vi "TestDataBase_1.vi"(9 "TableName":string="TestTable1", 10 "Select":string(combo)="Idle") -> (3 "ReadData":string[][](array[string]))   [LabVIEW 2024]
uses:
  Controls/Data_Cluster_TestDataBase.ctl
  Controls/DataBaseControl_Test.ctl
  <vilib>/addons/database/Auxilliary.llb/DB Tools Column Info.ctl
  <vilib>/addons/database/Auxilliary.llb/DB Tools DataTypes.ctl
  <vilib>/addons/database/Connection.llb/DB Tools Open Connec (String).vi
  <vilib>/addons/database/_DB Variant To Data/Database Variant To Data.xnode
  <vilib>/addons/database/NI_Database_API.lvlib
panel:
  out "time string":string
  out "date string":string
  out "concatenated string 2":string
  out "Select 2":string
  out "array":string[](array[string])
  out "String 2":string
  in  "Tab Control 2":enum32{"Page 1", "Page 2"}(tab)
  in  "BARCODE":string="1111"
  in  "Tab Control":enum32{"Page 1", "Page 2"}(tab)
  in  "Station4":T1={"BarCode"="1111", "Data1"="10", "Data2"="11", "Data3"="12"}
  in  "Station3":T1={"BarCode"="1111", "Data1"="7", "Data2"="8", "Data3"="9"}
  in  "Station2":T1={"BarCode"="1111", "Data1"="4", "Data2"="6", "Data3"="6"}
  in  "Station1":T1={"BarCode"="1112", "Data1"="1", "Data2"="2", "Data3"="3"}
  out "Date_Time":cluster{"Date":string, "Time":string}
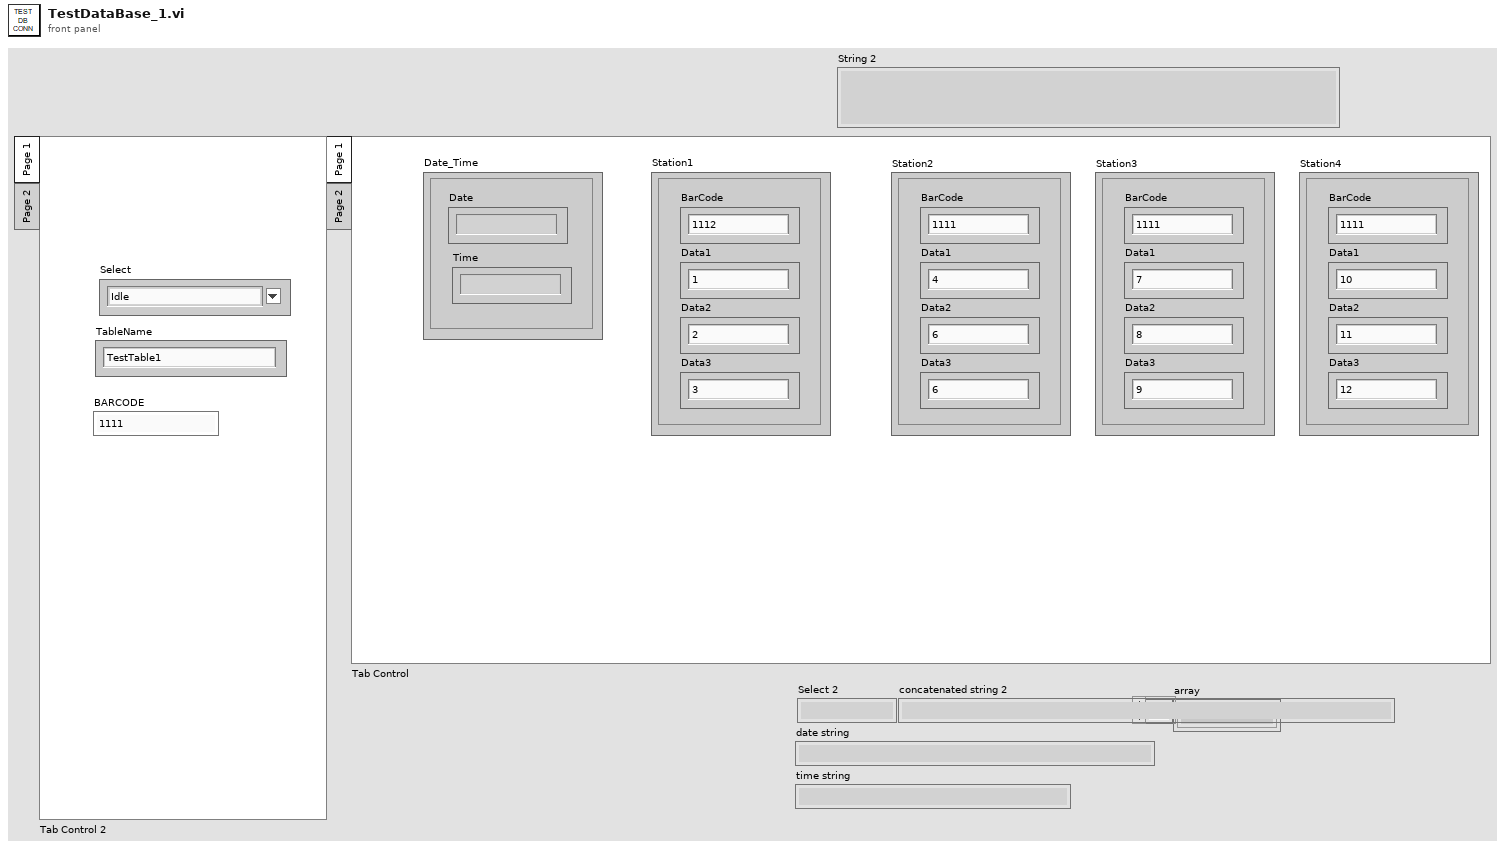
[diagram p1: front panel]
types:
  T1 = typedef "Data_Cluster_TestDataBase.ctl" = cluster{"BarCode":string, "Data1":string, "Data2":string, "Data3":string}
  T2 = typedef "DataBaseControl_Test.ctl" = cluster{"Date_Time":cluster{"Date":string, "Time":string}, "Station1":T1, "Station2":T1, "Station3":T1, "Station4":T1, "BARCODE":string, "ReadData":string[][]}
  T3 = typedef "NI_Database_API.lvlib/DB Tools Column Info.ctl" = cluster{"column name":string, "data type":T4, "size":i32, "allow null?":bool}
  T4 = typedef "NI_Database_API.lvlib/DB Tools DataTypes.ctl" = enum16{"String", "Long (I32)", "Single (SGL)", "Double (DBL)", "Date/Time", "Binary"}
  T5 = typedef "NI_Database_API.lvlib/Conn ObjectReference.ctl" = refnum<k1>
  T6 = cluster{"[0]":string, "[1]":string, "[2]":string, "[3]":string, "[4]":string, "[5]":string, "[6]":string, "[7]":string, "[8]":string, "[9]":string, "[10]":string, "[11]":string, "[12]":string, "[13]":string, "[14]":string, "[15]":string, "[16]":string, "[17]":string}
  T7 = cluster{"output array[0]":string, "output array[1]":string, "output array[2]":string, "output array[3]":string, "output array[4]":string, "output array[5]":string, "output array[6]":string, "output array[7]":string, "output array[8]":string, "output array[9]":string, "output array[10]":string, "output array[11]":string, "output array[12]":string, "output array[13]":string, "output array[14]":string, "output array[15]":string, "output array[16]":string, "output array[17]":string}
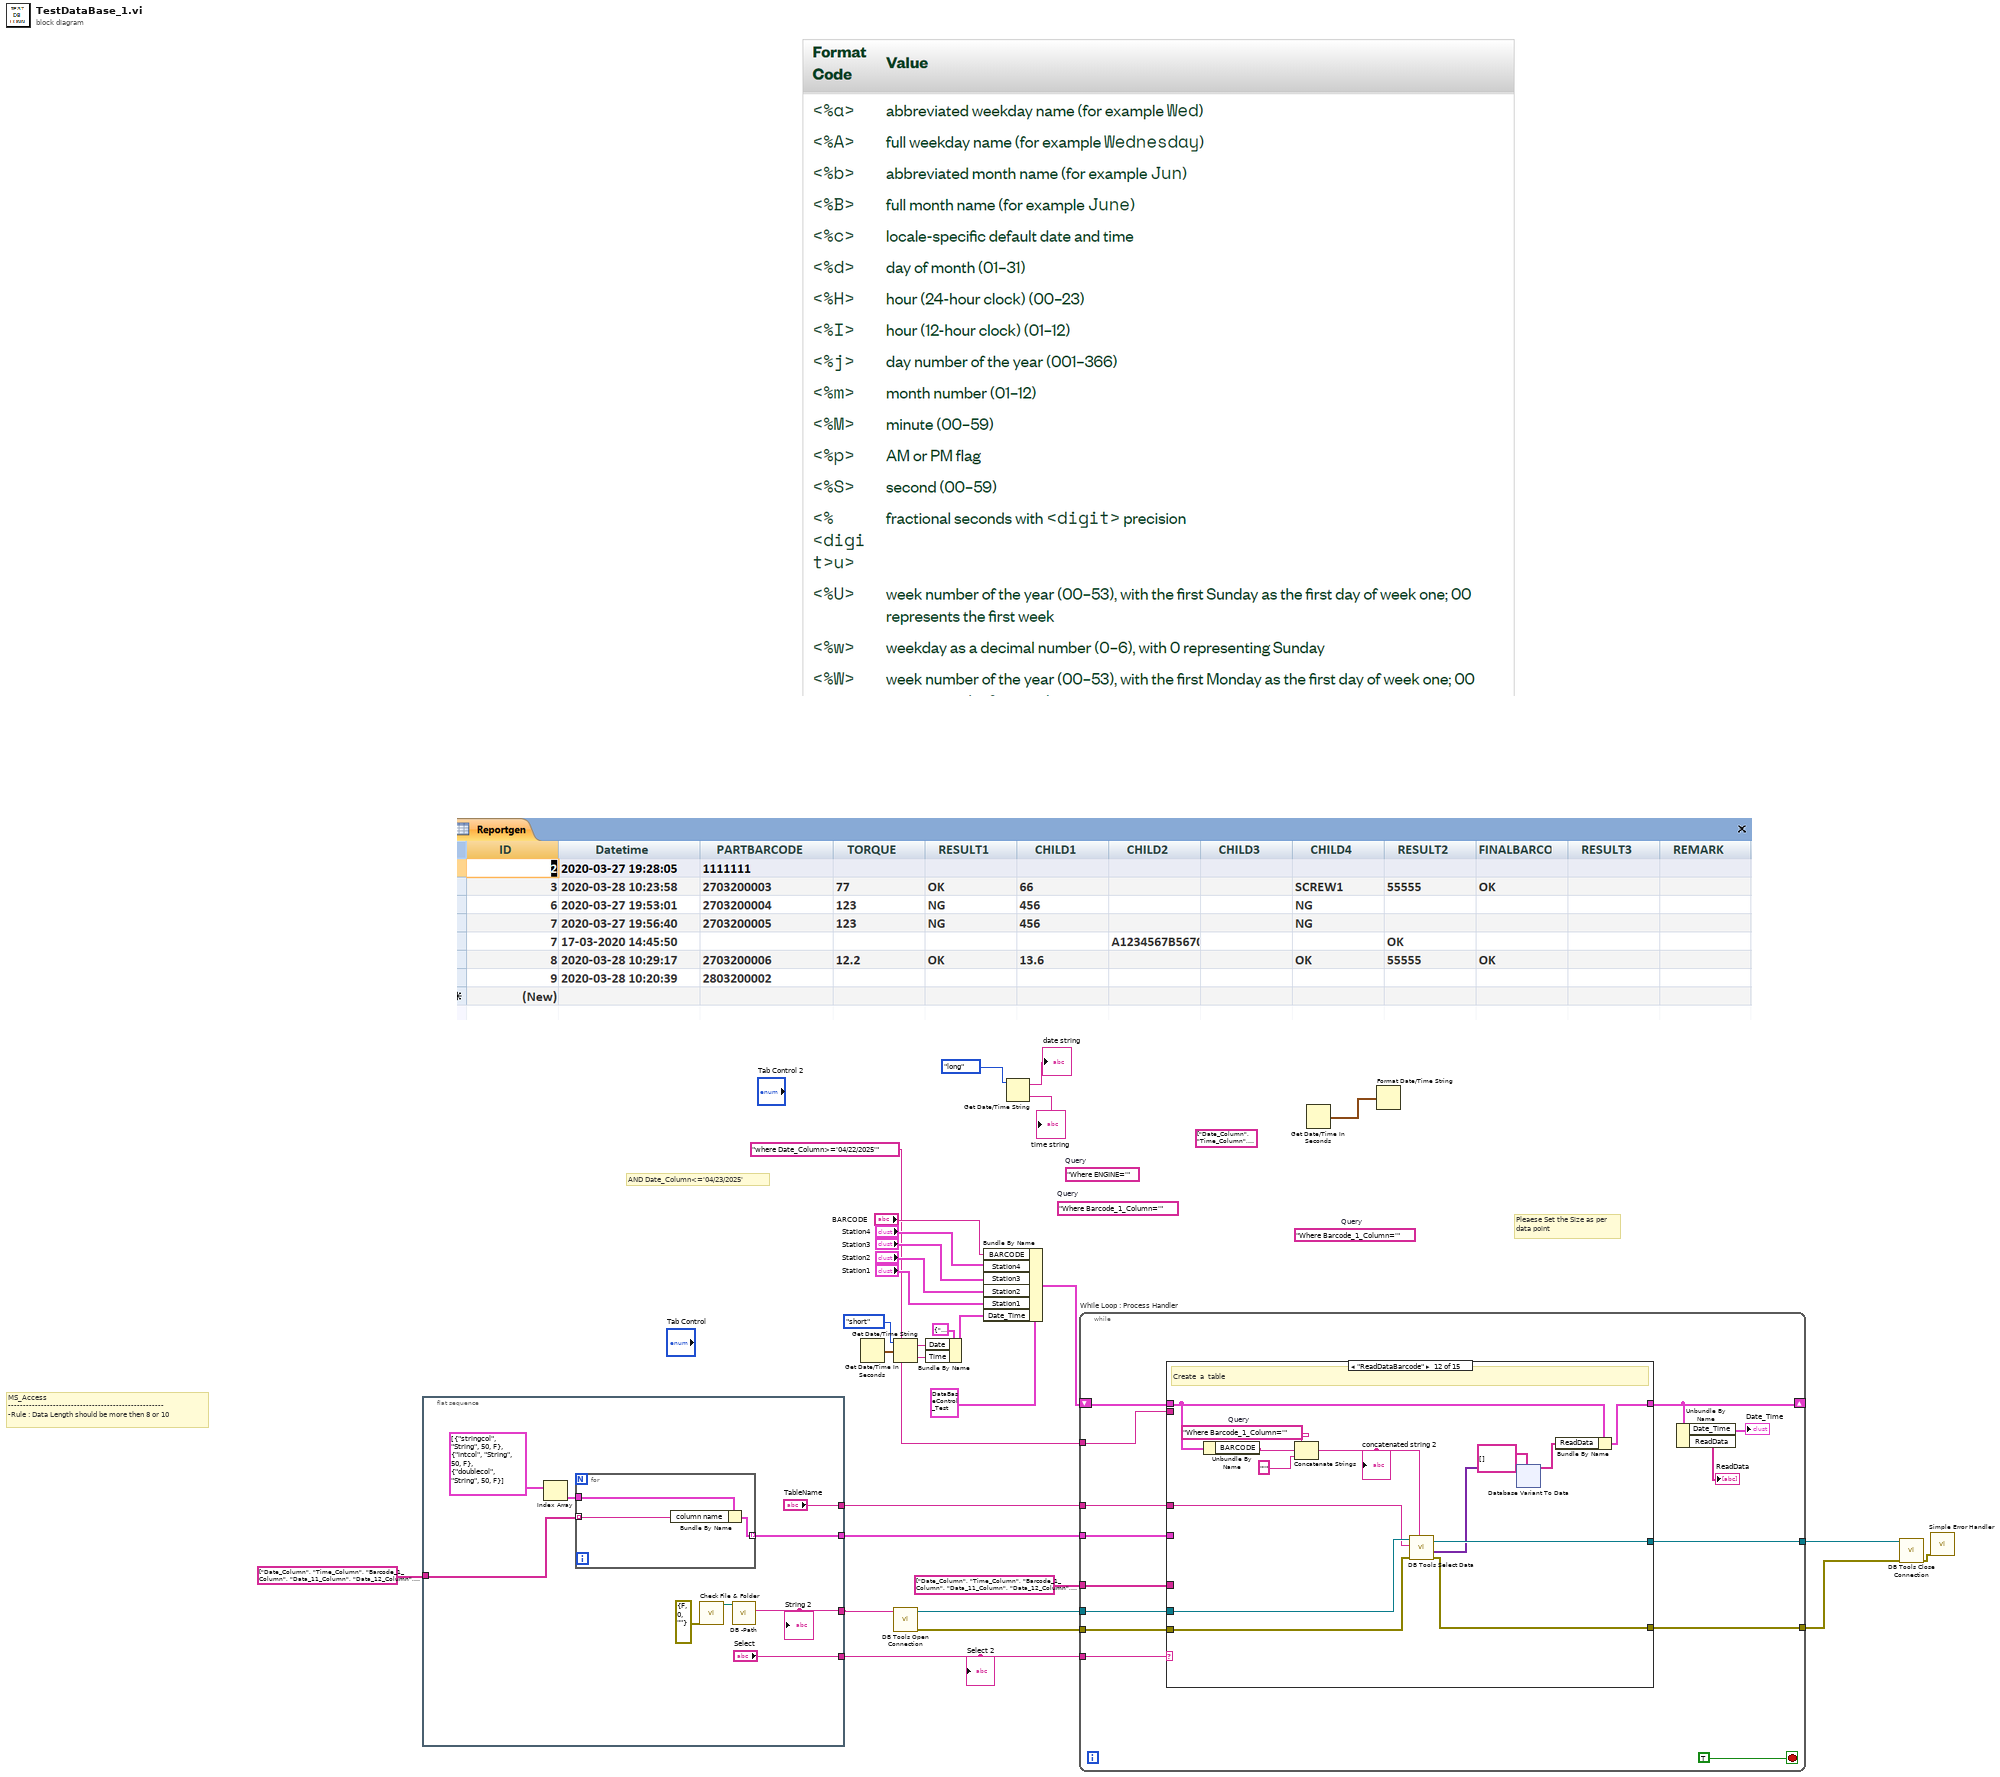
[diagram p0: block diagram]
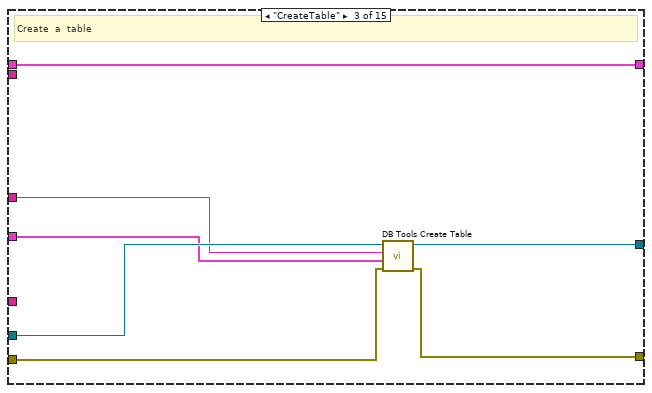
[diagram p4: hidden frame]
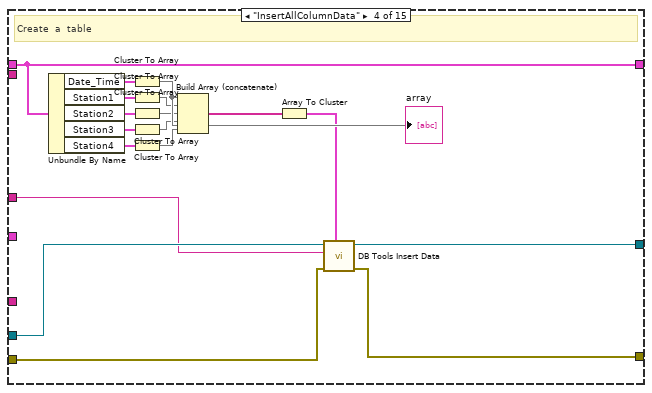
[diagram p5: hidden frame]
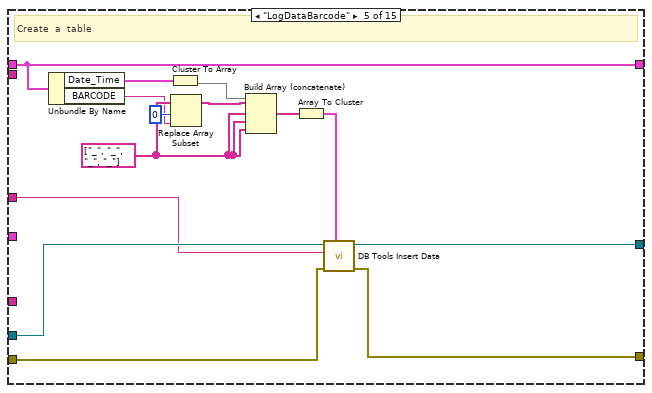
[diagram p6: hidden frame]
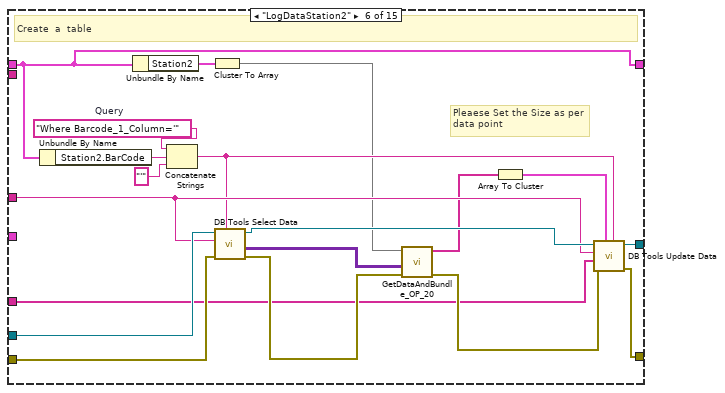
[diagram p7: hidden frame]
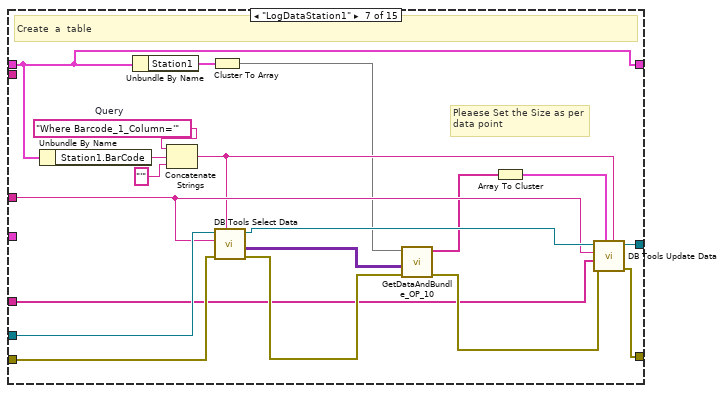
[diagram p8: hidden frame]
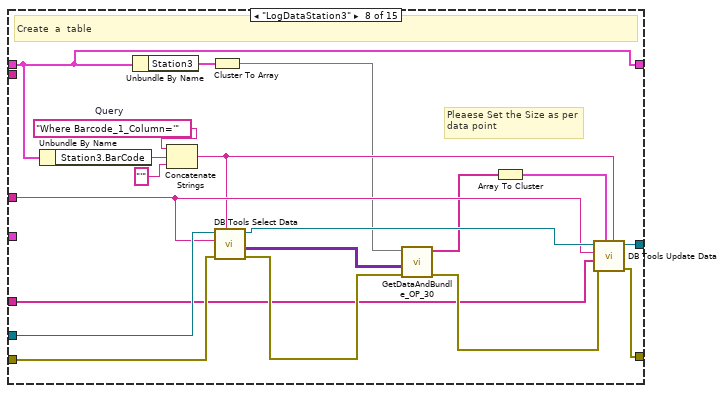
[diagram p9: hidden frame]
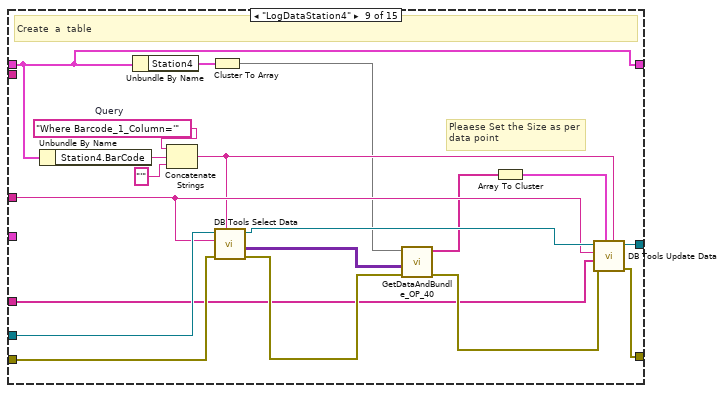
[diagram p10: hidden frame]
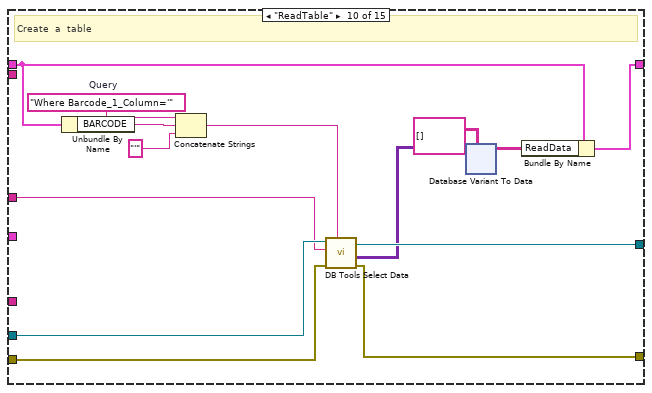
[diagram p11: hidden frame]
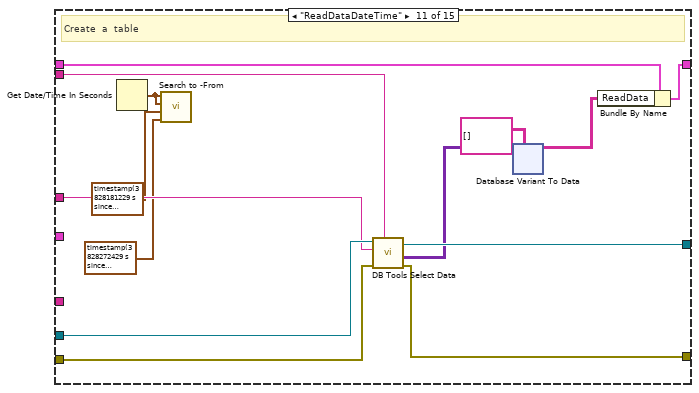
[diagram p12: hidden frame]
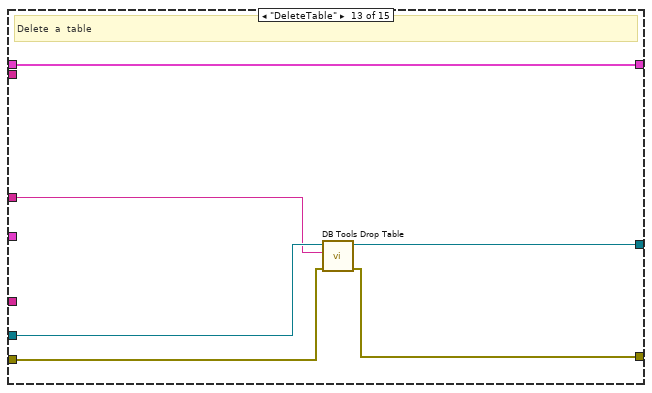
[diagram p13: hidden frame]
diagram:
  (unwired) string[] ["Date_Column", "Time_Column", "Barcode_1_Column", "Data_11_Column", "Data_12_Column", "Data_13_Column", "Barcode_2_Column", "Data_21_Column", "Data_22_Column", "Data_23_Column", "Barcode_3_Column", "Data_31_Column", "Data_32_Column", "Data_33_Column", "Barcode_4_Column", "Data_41_Column", "Data_42_Column", "Data_43_Column"] ("appended array")
  (unwired) "Where Barcode_1_Column='"  # Query
  (unwired) "Where Barcode_1_Column='"  # Query
  (unwired) "Where ENGINE='"  # Query
  # "AND Date_Column<='04/23/2025'"
  # "Pleaese Set the Size as per\ndata point"
  # "MS_Access \n----------------------------------------------------\n-Rule : Data Length should be more then 8 or 10"
  n1 = flat-sequence {
    tunnel: [w36] -> w29
    tunnel: ["Select"] -> w28
    tunnel: [w32] -> w22
    tunnel: string[] ["Date_Column", "Time_Column", "Barcode_1_Column", "Data_11_Column", "Data_12_Column", "Data_13_Column", "Barcode_2_Column", "Data_21_Column", "Data_22_Column", "Data_23_Column", "Barcode_3_Column", "Data_31_Column", "Data_32_Column", "Data_33_Column", "Barcode_4_Column", "Data_41_Column", "Data_42_Column", "Data_43_Column"] ("appended array") -> [w31]
    tunnel: ["TableName"] -> w20
    frame #0 {
      n2 = Index Array(array=T3[] [{"column name"="stringcol", "data type"=enum."String", "size"=50, "allow null?"=FALSE}, {"column name"="intcol", "data type"=enum."String", "size"=50, "allow null?"=FALSE}, {"column name"="doublecol", "data type"=enum."String", "size"=50, "allow null?"=FALSE}] ("column information")) -> (element=w34:T3)  [unwired: 1 in]
      n3 = for {
        tunnel: w34 -> [w41]
        tunnel: w31 -> [w40] mode=indexing
        tunnel: [w39] -> w32 mode=indexing
        n4 = Bundle By Name(cluster=w41, "column name"=w40) -> (w39:T3)
      }
      n5 = call "Check File & Folder .vi"("error in (no error)"=errorcluster {"status"=FALSE, "code"=0, "source"=""}) -> ("Config Path"=w37:path)  [unwired: 8 in, 2 out]
      n6 = call "DB -Path.vi"("path"=w37) -> ("String 2"=w36:string)  [unwired: 8 in, 2 out]
      "String 2" <- w36
    }
  }
  n7 = Get Date/Time In Seconds() -> (seconds since 1Jan1904=w17:timestamp)
  n8 = Get Date/Time String(date format (0)=enum16{"short", "long", "abbreviated"}."short", seconds (now)=w17) -> (date string=w16:string, time string=w15:string)  [unwired: 1 in]
  n9 = call-poly <vilib>:"DB Tools Open Connection.vi"("connection information"=w29) -> ("error out"=w27:errorcluster, "connection reference"=w26:T5)  [unwired: 7 in]
  n10 = Bundle By Name(cluster=cluster{"Date":string, "Time":string} {"Date"="", "Time"=""} ("Date_Time"), "Date"=w16, "Time"=w15) -> (w12:cluster{"Date":string, "Time":string})
  n11 = Bundle By Name(cluster=T2 {"Date_Time"={"Date"="4/19/2025", "Time"="9:54 PM"}, "Station1"={"BarCode"="1111", "Data1"="1", "Data2"="2", "Data3"="3"}, "Station2"={"BarCode"="1111", "Data1"="4", "Data2"="6", "Data3"="6"}, "Station3"={"BarCode"="1111", "Data1"="7", "Data2"="8", "Data3"="9"}, "Station4"={"BarCode"="1111", "Data1"="10", "Data2"="11", "Data3"="12"}, "BARCODE"="1111", "ReadData"=[]} ("Data_Cluster"), "BARCODE"="BARCODE", "Station4"="Station4", "Station3"="Station3", "Station2"="Station2", "Station1"="Station1", "Date_Time"=w12) -> (w18:T2)
  n12 = Get Date/Time String(date format (0)=enum16{"short", "long", "abbreviated"}."long") -> (date string=→"date string":string, time string=→"time string":string)  [unwired: 2 in]
  n13 = while "While Loop : Process Handler" {
    tunnel: w28 -> [w54]
    tunnel: w27 -> [w50]
    tunnel: w26 -> [w52]
    shift-right: [w46] -> _
    shift-left: w18 -> [w53]
    tunnel: w22 -> [w51]
    tunnel: [w49] -> w24
    tunnel: [w48] -> w23
    tunnel: w20 -> [w47]
    tunnel: string[] ["Date_Column", "Time_Column", "Barcode_1_Column", "Data_11_Column", "Data_12_Column", "Data_13_Column", "Barcode_2_Column", "Data_21_Column", "Data_22_Column", "Data_23_Column", "Barcode_3_Column", "Data_31_Column", "Data_32_Column", "Data_33_Column", "Barcode_4_Column", "Data_41_Column", "Data_42_Column", "Data_43_Column"] ("appended array") -> [w44]
    tunnel: "where Date_Column>='04/22/2025'" ("concatenated string") -> [w42]
    stop <- TRUE stop-if-true
    n14 = case shown="\"ReadDataBarcode\"" w54 {
      tunnel: w53 -> [w56 w61 w68 w82 w96 w114 w133 w152 w171 w179 w238 w295 w356 w359 w362]
      tunnel: [w56 w61 w68 w82 w96 w114 w133 w152 w171 w177 w237 w294 w356 w359 w362] -> w46
      tunnel: w52 -> [w58 w60 w67 w86 w100 w119 w138 w157 w176 w186 w246 w302 w355 w358 w361]
      tunnel: w51 -> [_ _ w63 _ _ _ _ _ _ _ _ _ _ _ _]
      tunnel: w50 -> [w57 w59 w66 w85 w99 w118 w137 w156 w175 w188 w248 w304 w354 w357 w360]
      tunnel: [w58 w60 w65 w84 w98 w108 w127 w146 w165 w183 w244 w299 w353 w358 w361] -> w49
      tunnel: [w57 w59 w64 w83 w97 w112 w131 w150 w169 w187 w247 w303 w352 w357 w360] -> w48
      tunnel: w47 -> [_ _ w62 w69 w92 w110 w129 w148 w167 w185 w245 w301 w351 _ _]
      tunnel: w44 -> [_ _ _ _ _ w101 w120 w139 w158 _ _ _ _ _ _]
      tunnel: w42 -> [_ _ _ _ _ _ _ _ _ _ w235 _ _ _ _]
      frame "Idle", Default {
      }
      frame "1--------------------------------------" {
        # "Delete  a  table"
      }
      frame "CreateTable" {
        # "Create  a  table"
        n15 = call <vilib>:"DB Tools Create Table.vi"("error in (no error)"=w66, "column information"=w63, "table"=w62, "connection reference"=w67) -> ("error out"=w64:errorcluster, "connection reference out"=w65:T5)  [unwired: 4 in]
      }
      frame "InsertAllColumnData" {
        # "Create  a  table"
        n16 = Unbundle By Name(w82) -> ("Date_Time"=w81:cluster{"Date":string, "Time":string}, "Station1"=w80:T1, "Station2"=w79:T1, "Station3"=w78:T1, "Station4"=w77:T1)
        n17 = Cluster To Array(cluster=w81) -> (array=w76:string[])
        "array" <- w76
        n18 = Cluster To Array(cluster=w80) -> (array=w75:string[])
        n19 = Cluster To Array(cluster=w79) -> (array=w74:string[])
        n20 = Cluster To Array(cluster=w78) -> (array=w73:string[])
        n21 = Cluster To Array(cluster=w77) -> (array=w72:string[])
        n22 = Build Array (concatenate)(w76, w75, w74, w73, w72) -> (w70:string[])
        n23 = Array To Cluster(array=w70) -> (cluster=w71:T6)
        n24 = call <vilib>:"DB Tools Insert Data.vi"("data"=w71, "error in (no error)"=w85, "table"=w69, "connection reference"=w86) -> ("error out"=w83:errorcluster, "connection reference out"=w84:T5)  [unwired: 6 in]
      }
      frame "LogDataBarcode" {
        w90 = string[] ["_", "_", "_", "_"]
        # "Create  a  table"
        n25 = Unbundle By Name(w96) -> ("Date_Time"=w95:cluster{"Date":string, "Time":string}, "BARCODE"=w88:string)
        n26 = Cluster To Array(cluster=w95) -> (array=w94:string[])
        n27 = Replace Array Subset(array=w90, new element=w88, index=0) -> (w87:string[])
        n28 = Build Array (concatenate)(w94, w87, w90, w90, w90) -> (w93:string[])
        n29 = Array To Cluster(array=w93) -> (cluster=w91:T6)
        n30 = call <vilib>:"DB Tools Insert Data.vi"("data"=w91, "error in (no error)"=w99, "table"=w92, "connection reference"=w100) -> ("error out"=w97:errorcluster, "connection reference out"=w98:T5)  [unwired: 6 in]
      }
      frame "LogDataStation2" {
        w115 = "Where Barcode_1_Column='"  # Query
        # "Pleaese Set the Size as per\ndata point"
        # "Create  a  table"
        n31 = Unbundle By Name(w114) -> ("Station2.BarCode"=w116:string)
        n32 = Unbundle By Name(w114) -> ("Station2"=w113:T1)
        n33 = Concatenate Strings(w115, w116, "'" ("string")) -> (w109:string)
        n34 = Cluster To Array(cluster=w113) -> (array=w106:string[])
        n35 = call <vilib>:"DB Tools Select Data.vi"("condition"=w109, "error in (no error)"=w118, "table"=w110, "connection reference"=w119) -> ("error out"=w104:errorcluster, "data"=w105:variant[][], "connection reference out"=w111:T5)  [unwired: 2 in]
        n36 = call "GetDataAndBundle_OP_20.vi"("error in (no error)"=w104, "data in"=w105, "StaionDataIn"=w106) -> ("error out"=w103:errorcluster, "output array"=w102:string[])  [unwired: 7 in]
        n37 = Array To Cluster(array=w102) -> (cluster=w107:T7)
        n38 = call <vilib>:"DB Tools Update Data.vi"("condition"=w109, "data"=w107, "error in (no error)"=w103, "columns"=w101, "table"=w110, "connection reference"=w111) -> ("error out"=w112:errorcluster, "connection reference out"=w108:T5)  [unwired: 4 in]
      }
      frame "LogDataStation1" {
        w134 = "Where Barcode_1_Column='"  # Query
        # "Pleaese Set the Size as per\ndata point"
        # "Create  a  table"
        n39 = Unbundle By Name(w133) -> ("Station1.BarCode"=w135:string)
        n40 = Unbundle By Name(w133) -> ("Station1"=w132:T1)
        n41 = Concatenate Strings(w134, w135, "'" ("string")) -> (w128:string)
        n42 = Cluster To Array(cluster=w132) -> (array=w125:string[])
        n43 = call <vilib>:"DB Tools Select Data.vi"("condition"=w128, "error in (no error)"=w137, "table"=w129, "connection reference"=w138) -> ("error out"=w123:errorcluster, "data"=w124:variant[][], "connection reference out"=w130:T5)  [unwired: 2 in]
        n44 = call "GetDataAndBundle_OP_10.vi"("error in (no error)"=w123, "data in"=w124, "StaionDataIn"=w125) -> ("error out"=w122:errorcluster, "output array"=w121:string[])  [unwired: 7 in]
        n45 = Array To Cluster(array=w121) -> (cluster=w126:T7)
        n46 = call <vilib>:"DB Tools Update Data.vi"("condition"=w128, "data"=w126, "error in (no error)"=w122, "columns"=w120, "table"=w129, "connection reference"=w130) -> ("error out"=w131:errorcluster, "connection reference out"=w127:T5)  [unwired: 4 in]
      }
      frame "LogDataStation3" {
        w153 = "Where Barcode_1_Column='"  # Query
        # "Pleaese Set the Size as per\ndata point"
        # "Create  a  table"
        n47 = Unbundle By Name(w152) -> ("Station3.BarCode"=w154:string)
        n48 = Unbundle By Name(w152) -> ("Station3"=w151:T1)
        n49 = Concatenate Strings(w153, w154, "'" ("string")) -> (w147:string)
        n50 = Cluster To Array(cluster=w151) -> (array=w144:string[])
        n51 = call <vilib>:"DB Tools Select Data.vi"("condition"=w147, "error in (no error)"=w156, "table"=w148, "connection reference"=w157) -> ("error out"=w142:errorcluster, "data"=w143:variant[][], "connection reference out"=w149:T5)  [unwired: 2 in]
        n52 = call "GetDataAndBundle_OP_30.vi"("error in (no error)"=w142, "data in"=w143, "StaionDataIn"=w144) -> ("error out"=w141:errorcluster, "output array"=w140:string[])  [unwired: 7 in]
        n53 = Array To Cluster(array=w140) -> (cluster=w145:T7)
        n54 = call <vilib>:"DB Tools Update Data.vi"("condition"=w147, "data"=w145, "error in (no error)"=w141, "columns"=w139, "table"=w148, "connection reference"=w149) -> ("error out"=w150:errorcluster, "connection reference out"=w146:T5)  [unwired: 4 in]
      }
      frame "LogDataStation4" {
        w172 = "Where Barcode_1_Column='"  # Query
        # "Pleaese Set the Size as per\ndata point"
        # "Create  a  table"
        n55 = Unbundle By Name(w171) -> ("Station4.BarCode"=w173:string)
        n56 = Unbundle By Name(w171) -> ("Station4"=w170:T1)
        n57 = Concatenate Strings(w172, w173, "'" ("string")) -> (w166:string)
        n58 = Cluster To Array(cluster=w170) -> (array=w163:string[])
        n59 = call <vilib>:"DB Tools Select Data.vi"("condition"=w166, "error in (no error)"=w175, "table"=w167, "connection reference"=w176) -> ("error out"=w161:errorcluster, "data"=w162:variant[][], "connection reference out"=w168:T5)  [unwired: 2 in]
        n60 = call "GetDataAndBundle_OP_40.vi"("error in (no error)"=w161, "data in"=w162, "StaionDataIn"=w163) -> ("error out"=w160:errorcluster, "output array"=w159:string[])  [unwired: 7 in]
        n61 = Array To Cluster(array=w159) -> (cluster=w164:T7)
        n62 = call <vilib>:"DB Tools Update Data.vi"("condition"=w166, "data"=w164, "error in (no error)"=w160, "columns"=w158, "table"=w167, "connection reference"=w168) -> ("error out"=w169:errorcluster, "connection reference out"=w165:T5)  [unwired: 4 in]
      }
      frame "ReadTable" {
        w189 = "Where Barcode_1_Column='"  # Query
        # "Create  a  table"
        n63 = Unbundle By Name(w179) -> ("BARCODE"=w180:string)
        n64 = Concatenate Strings(w189, w180, "'" ("string")) -> (w184:string)
        n65 = call <vilib>:"DB Tools Select Data.vi"("condition"=w184, "error in (no error)"=w188, "table"=w185, "connection reference"=w186) -> ("error out"=w187:errorcluster, "data"=w181:variant[][], "connection reference out"=w183:T5)  [unwired: 2 in]
        n66 = xnode "Database Variant To Data"("database variant"=w181, "type"=string[][] []) -> ("data"=w178:string[][])  [unwired: 1 in, 1 out]
        n67 = Bundle By Name(cluster=w179, "ReadData"=w178) -> (w177:T2)
      }
      frame "ReadDataDateTime" {
        # "Create  a  table"
        n68 = Get Date/Time In Seconds() -> (seconds since 1Jan1904=w240:timestamp)
        n69 = call "Search to -From.vi"("EndDate"=timestamp(3828272429.0624337 s since 1904-01-01), "StartDate"=timestamp(3828181229.0624337 s since 1904-01-01), "From date"=w240, "To Date"=w240) -> ()  [unwired: 6 in, 2 out]
        n70 = call <vilib>:"DB Tools Select Data.vi"("condition"=w235, "error in (no error)"=w248, "table"=w245, "connection reference"=w246) -> ("error out"=w247:errorcluster, "data"=w242:variant[][], "connection reference out"=w244:T5)  [unwired: 2 in]
        n71 = xnode "Database Variant To Data"("database variant"=w242, "type"=string[][] []) -> ("data"=w236:string[][])  [unwired: 1 in, 1 out]
        n72 = Bundle By Name(cluster=w238, "ReadData"=w236) -> (w237:T2)
      }
      frame "ReadDataBarcode" {
        w305 = "Where Barcode_1_Column='"  # Query
        # "Create  a  table"
        n73 = Unbundle By Name(w295) -> ("BARCODE"=w296:string)
        n74 = Concatenate Strings(w305, w296, "'" ("string")) -> (w300:string)
        "concatenated string 2" <- w300
        n75 = call <vilib>:"DB Tools Select Data.vi"("condition"=w300, "error in (no error)"=w304, "table"=w301, "connection reference"=w302) -> ("error out"=w303:errorcluster, "data"=w297:variant[][], "connection reference out"=w299:T5)  [unwired: 2 in]
        n76 = xnode "Database Variant To Data"("database variant"=w297, "type"=string[][] []) -> ("data"=w293:string[][])  [unwired: 1 in, 1 out]
        n77 = Bundle By Name(cluster=w295, "ReadData"=w293) -> (w294:T2)
      }
      frame "DeleteTable" {
        # "Delete  a  table"
        n78 = call <vilib>:"DB Tools Drop Table.vi"("error in (no error)"=w354, "table"=w351, "connection reference"=w355) -> ("error out"=w352:errorcluster, "connection reference out"=w353:T5)  [unwired: 5 in]
      }
      frame "2--------------------------------------" {
        # "Delete  a  table"
      }
      frame "3--------------------------------------" {
        # "Delete  a  table"
      }
    }
    n79 = Unbundle By Name(w46) -> ("Date_Time"=→"Date_Time":cluster{"Date":string, "Time":string}, "ReadData"=→"ReadData":string[][])
  }
  n80 = Get Date/Time In Seconds() -> (seconds since 1Jan1904=w1:timestamp)
  n81 = Format Date/Time String(seconds (now)=w1) -> ()  [unwired: 2 in, 1 out]
  n82 = call <vilib>:"DB Tools Close Connection.vi"("error in (no error)"=w23, "connection reference"=w24) -> ("error out"=w25:errorcluster)  [unwired: 5 in]
  n83 = call <vilib>:"Simple Error Handler.vi"("error in (no error)"=w25) -> ()  [unwired: 4 in, 5 out]
  "Select 2" <- w28
